vi "UDP dSpace Reveiver.vi"(7 "milliseconds to wait":u32, 8 "error in (no error)":errorcluster, 10 "ENQUE DIRECTLY":refnum<queue>, 11 "UDP Network Connection in":refnum<k16>) -> (0 "error out":errorcluster)   [LabVIEW 2016]
uses:
  Globale Variablen VI/AutonomousMode.vi
  Globale Variablen VI/Global Variables.vi
panel:
  out "value":u32
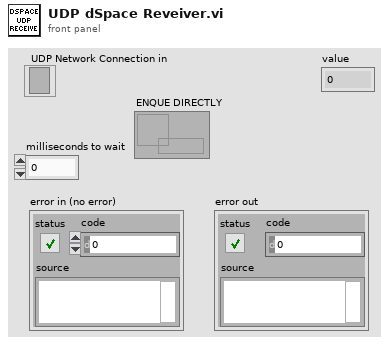
[diagram p1: front panel]
types:
  T1 = enum16{"big-endian, network order", "native, host order", "little-endian"}
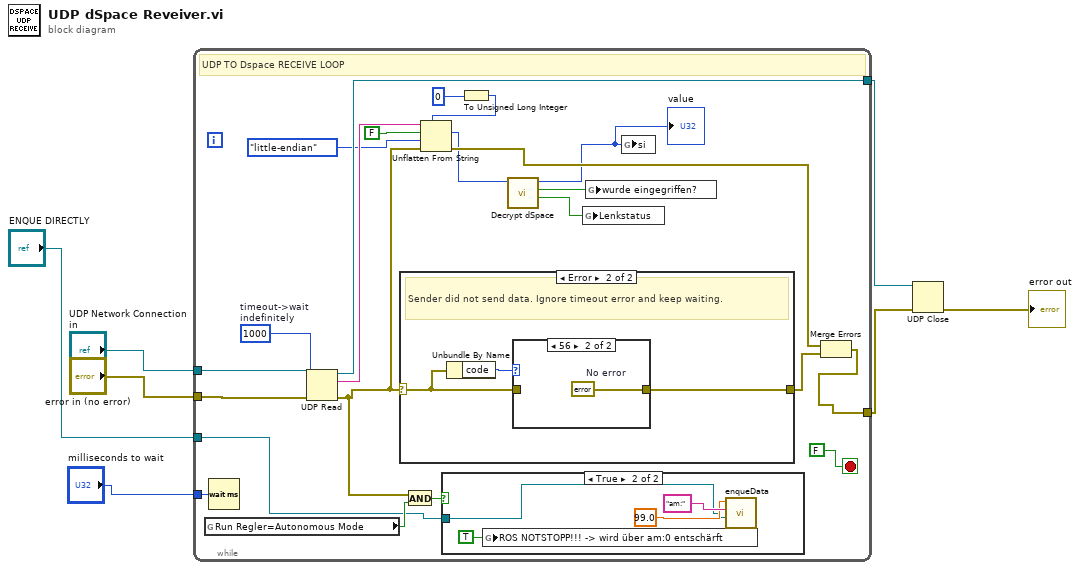
[diagram p0: block diagram]
diagram:
  n1 = while {
    tunnel: [w29] -> w5
    tunnel: [w19] -> w6
    tunnel: "UDP Network Connection in" -> [w27]
    tunnel: "error in (no error)" -> [w26]
    tunnel: "milliseconds to wait" -> [w18]
    tunnel: "ENQUE DIRECTLY" -> [w9]
    stop <- FALSE stop-if-true
    w28 = 1000  # timeout->wait indefinitely
    # "UDP TO Dspace RECEIVE LOOP"
    n2 = global read "AutonomousMode.vi" "Run Regler=Autonomous Mode"() -> (w12:bool)
    n3 = Wait (ms)(milliseconds to wait=w18) -> ()  [unwired: 1 out]
    n4 = UDP Read(connection ID=w27, timeout ms (25000)=w28, 8:w26) -> (data out=w25:string, error out=w11:errorcluster, 3:w29:refnum<k16>)  [unwired: 3 out]
    n5 = case shown="Error" w11 {
      selector: w11 -> [w34 w36]
      tunnel: [w34 w35] -> w20
      frame No Error {
        # "Sender sent data. Update the chart value."
      }
      frame Error {
        # "Sender did not send data. Ignore timeout error and keep waiting."
        n6 = Unbundle By Name(w36) -> ("code"=w37:i32)
        n7 = case shown="56" w37 {
          tunnel: w36 -> [w38 _]
          tunnel: [w38 w39] -> w35
          frame Default {
          }
          frame 56 {
            w39 = errorcluster {"status"=FALSE, "code"=0, "source"=""}  # No error
          }
        }
      }
    }
    n8 = And(x=w11, y=w12) -> (x .and. y?=w10:bool)
    n9 = case shown="True" w10 {
      tunnel: w9 -> [_ w30]
      frame False {
      }
      frame True {
        n10 = global write "AutonomousMode.vi" "ROS NOTSTOPP!!! -> wird über am:0 entschärft"(TRUE ("ROS NOTSTOPP!!! -> wird über am:0 entschärft")) -> ()
        n11 = call "enqueData.vi"("Queue Reference"=w30, "Descriptor"="am:", "Value IN"=99.0) -> ()  [unwired: 8 in, 1 out]
      }
    }
    n12 = To Unsigned Long Integer(number=0) -> (unsigned 32bit integer=w21:u32)
    n13 = Unflatten From String(type=w21, binary string=w25, data includes array or string size? (T)=FALSE, byte order (0:big-endian, network order)=T1."little-endian", error in (no error)=w11) -> (value=w16:u32, error out=w17:errorcluster)  [unwired: 1 out]
    n14 = call "Decrypt dSpace.vi"("Numeric in"=w16) -> ("Lenkstatus"=w13:bool, "wurde eingegriffen?"=w14:bool, "Numeric out"=w15:u32)  [unwired: 8 in]
    "value" <- w15
    n15 = global write "Global Variables.vi" "Lenkstatus"(w13) -> ()
    n16 = global write "Global Variables.vi" "wurde eingegriffen?"(w14) -> ()
    n17 = global write "Global Variables.vi" "si"(w15) -> ()
    n18 = Merge Errors(w17, w20) -> (w19:errorcluster)
  }
  n19 = UDP Close(connection ID=w5, 8:w6) -> (error out=→"error out":errorcluster)  [unwired: 1 out]
